vi "Shoot.vi"(1 "millisecond timer value":u32, 2 "Shoot":bool=TRUE) -> ()   [LabVIEW 2016]
uses:
  <vilib>/Rock Robotics/WPI/SafetyOutput/WPI_SafetyOutputConfigMenu.ctl
  Global 2.vi
  <vilib>/gmath/NI_Gmath.lvlib
panel:
  in  "Adjustment X":dbl[](array[numeric])=[-3400.0, -3100.0, -2750.0, -2430.0, -2080.0, -1710.0, -1330.0, -950.0, -580.0, -210.0, 0.0, 210.0, 580.0, 950.0, 1330.0, 1710.0, 2080.0, 2430.0, 2750.0, 3100.0, 3400.0]
  in  "Adjustment Y":dbl[](array[numeric])=[-1.0, -0.9, -0.8, -0.7, -0.6, -0.5, -0.4, -0.3, -0.2, -0.1, 0.0, 0.1, 0.2, 0.3, 0.4, 0.5, 0.6, 0.7, 0.8, 0.9, 1.0] format="%_6g"
  out "Waveform Chart":cluster{dbl}(graph)={2565.46875}
  out "Motor Effort":dbl=0.17108041660508766
  out "Adjustment":dbl=-0.27365642550017555
  out "RPM":dbl=2565.46875
  in  "kP":dbl=0.8 format="%#_13g"
  in  "kD":dbl=0.06 format="%#_13g"
  in  "Y":dbl[](array[numeric])=[0.0, 0.1, 0.2, 0.3, 0.4, 0.5, 0.6, 0.7, 0.8, 0.9, 1.0] format="%_6g"
  in  "X":dbl[](array[numeric])=[0.0, 210.0, 580.0, 950.0, 1330.0, 1710.0, 2080.0, 2430.0, 2750.0, 3100.0, 3400.0]
  in  "RPM Target BB":dbl=1500.0
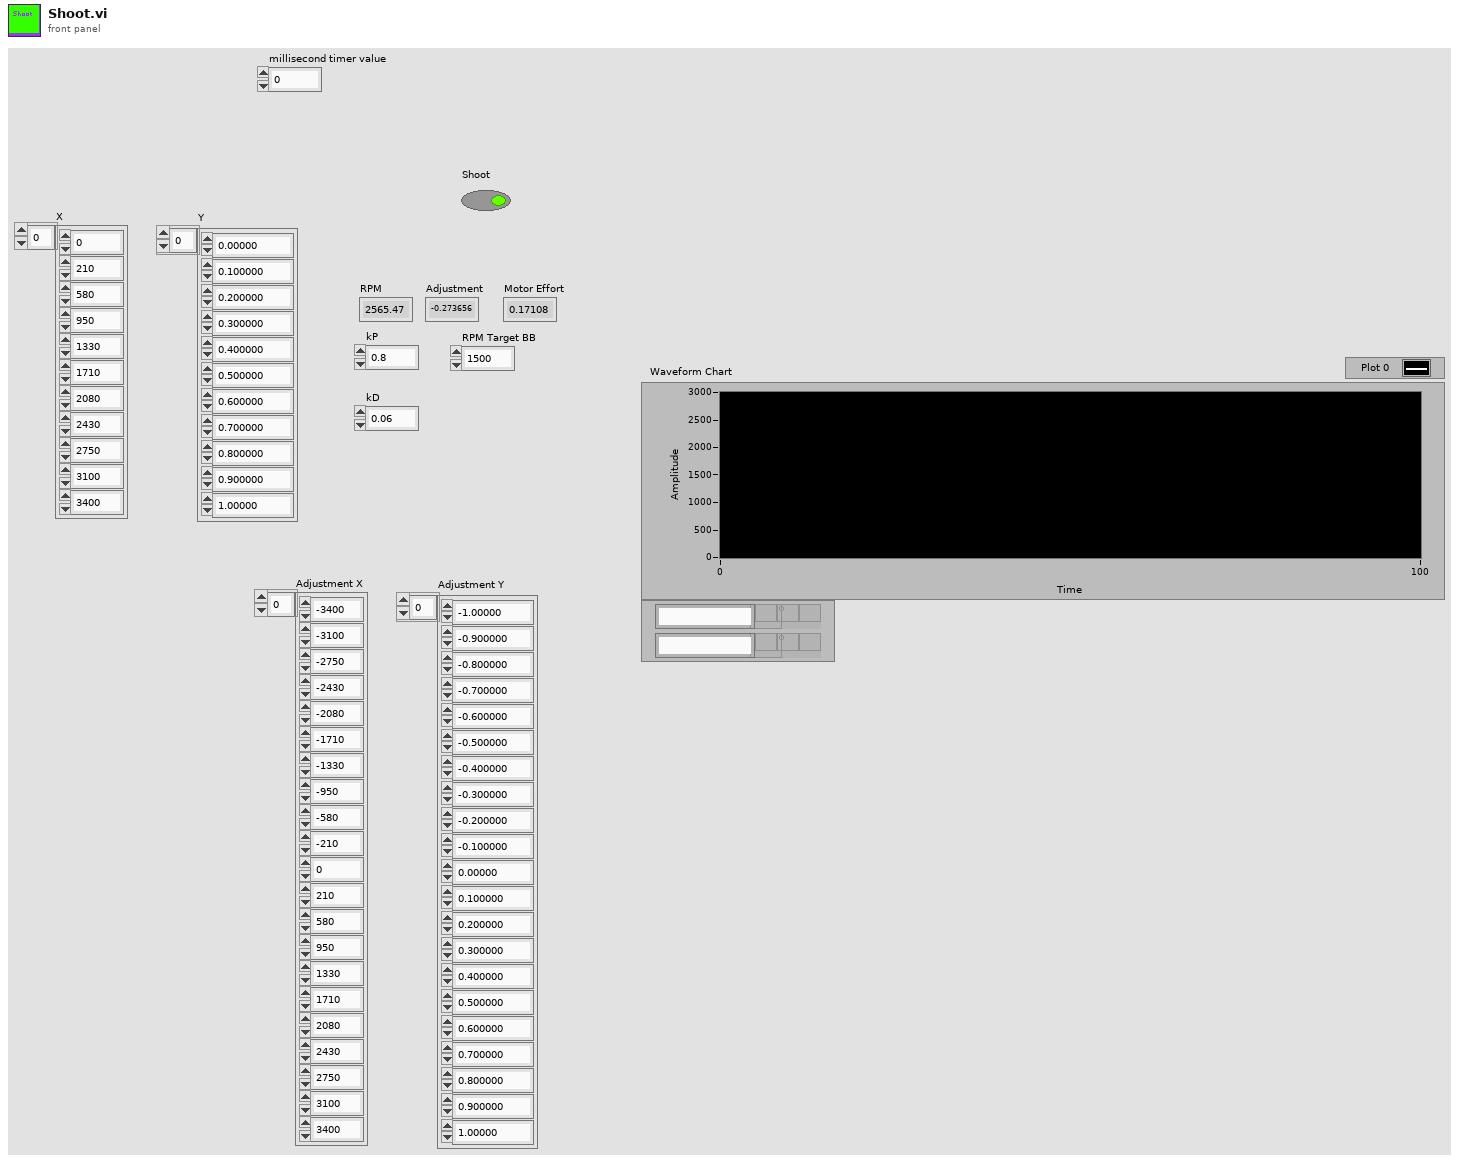
[diagram p1: front panel]
types:
  T1 = typedef "WPI_SafetyOutputConfigMenu.ctl" = enum16{"Enable", "Disable"}
  T2 = typedef "WPI_MotorControlDeviceRef.ctl" = cluster{"DeviceStatus":errorcluster, "Type":T3, "PWM":cluster{"PWM Channel":T4, "DeadBand":T5}, "CAN":cluster{"Device Number":u8, "SetOutput VI Ref":variant, "GetOutput VI Ref":variant, "Enable VI Ref":variant, "Disable VI Ref":variant, "Data":variant}, "Invert":bool}
  T3 = typedef "WPI_MotorControlType.ctl" = enum16{"PWM", "CAN"}
  T4 = typedef "FPGA_DIOPWMChannel.ctl" = enum8{"PWM 0", "PWM 1", "PWM 2", "PWM 3", "PWM 4", "PWM 5", "PWM 6", "PWM 7", "PWM 8", "PWM 9", "PWM MXP 0", "PWM MXP 1", "PWM MXP 2", "PWM MXP 3", "PWM MXP 4", "PWM MXP 5", "PWM MXP 6", "PWM MXP 7", "PWM MXP 8", "PWM MXP 9", "Invalid"}
  T5 = typedef "WPI_PWMDeadband.ctl" = cluster{"Name":string, "maxPositivePwm":i32, "minPositivePwm":i32, "centerPwm":i32, "maxNegativePwm":i32, "minNegativePwm":i32, "angularRange":u16}
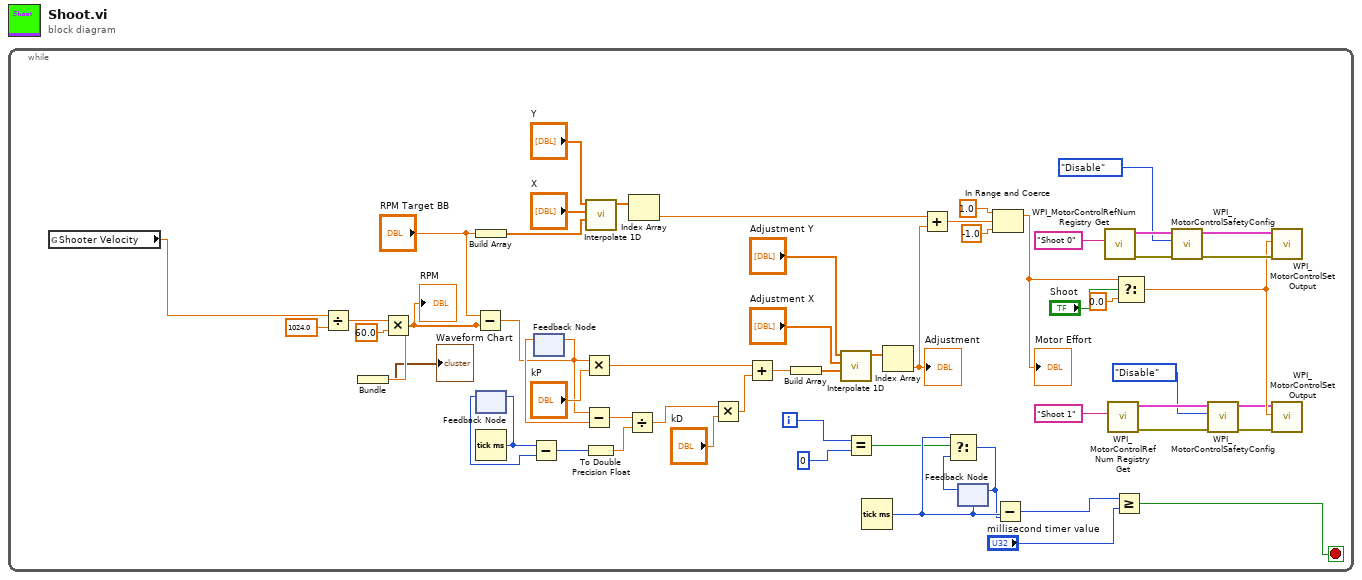
[diagram p0: block diagram]
diagram:
  n1 = while {
    i -> [w4]
    stop <- w1 stop-if-true
    n2 = global read "Global 2.vi" "Shooter Velocity"() -> (w21:dbl)
    n3 = Divide(x=w21, y=1024.0) -> (x/y=w56:dbl)
    n4 = Multiply(x=w56, y=60.0) -> (x*y=w27:dbl)
    "RPM" <- w27
    n5 = Bundle(w27) -> (→"Waveform Chart":cluster{dbl})  [unwired: 1 in]
    n6 = Subtract(x="RPM Target BB", y=w27) -> (x-y=w29:dbl)
    n7 = Build Array("RPM Target BB") -> (w54:dbl[])
    n8 = feedback #1() -> (w50:u32)  [unwired: 1 in]
    n9 = Tick Count (ms)() -> (millisecond timer value=w51:u32)
    n10 = feedback-in #1(w51) -> ()
    n11 = Subtract(x=w51, y=w50) -> (x-y=w48:u32)
    n12 = feedback #2() -> (w52:dbl)  [unwired: 1 in]
    n13 = feedback-in #2(w29) -> ()
    n14 = Multiply(x=w29, y="kP") -> (x*y=w42:dbl)
    n15 = Subtract(x=w29, y=w52) -> (x-y=w49:dbl)
    n16 = call <vilib>:"Interpolate 1D.vi"("xi"=w54, "X"="X", "Y"="Y") -> ("yi"=w53:dbl[])  [unwired: 6 in, 2 out]
    n17 = To Double Precision Float(number=w48) -> (double precision float=w47:dbl)
    n18 = Divide(x=w49, y=w47) -> (x/y=w46:dbl)
    n19 = Index Array(array=w53) -> (element=w40:dbl)  [unwired: 1 in]
    n20 = Multiply(x=w46, y="kD") -> (x*y=w41:dbl)
    n21 = Add(x=w42, y=w41) -> (x+y=w35:dbl)
    n22 = Build Array(w35) -> (w38:dbl[])
    n23 = call <vilib>:"Interpolate 1D.vi"("xi"=w38, "X"="Adjustment X", "Y"="Adjustment Y") -> ("yi"=w39:dbl[])  [unwired: 6 in, 2 out]
    n24 = Equal?(x=w4, y=0) -> (x = y?=w7:bool)
    n25 = Tick Count (ms)() -> (millisecond timer value=w9:u32)
    n26 = Index Array(array=w39) -> (element=w34:dbl)  [unwired: 1 in]
    "Adjustment" <- w34
    n27 = Add(x=w40, y=w34) -> (x+y=w33:dbl)
    n28 = feedback #3(w9) -> (w8:u32)
    n29 = Select(t=w9, s=w7, f=w8) -> (s? t:f=w5:u32)
    n30 = feedback-in #3(w5) -> ()
    n31 = In Range and Coerce(upper limit=1.0, x=w33, lower limit=-1.0 ("upper limit")) -> (coerced(x)=w30:dbl)  [unwired: 1 out]
    "Motor Effort" <- w30
    n32 = Subtract(x=w9, y=w5) -> (x-y=w3:u32)
    n33 = call <vilib>:"WPI_MotorControlRefNum Registry Get.vi"("refnum name"="Shoot 0") -> ("error out"=w10:errorcluster, "MotorControlDevRef"=w20:T2)  [unwired: 9 in]
    n34 = call <vilib>:"WPI_MotorControlRefNum Registry Get.vi"("refnum name"="Shoot 1") -> ("error out"=w15:errorcluster, "MotorControlDevRef"=w16:T2)  [unwired: 9 in]
    n35 = Greater Or Equal?(x=w3, y="millisecond timer value") -> (x >= y?=w1:bool)
    n36 = Select(t=w30, s="Shoot", f=0.0) -> (s? t:f=w14:dbl)
    n37 = call <vilib>:"WPI_MotorControlSafetyConfig.vi"("error in (no error)"=w10, "mode"=WPI_SafetyOutputConfigMenu."Disable", "MotorControlDevRef"=w20) -> ("error out"=w18:errorcluster, "MotorControlDevRef"=w19:T2)  [unwired: 7 in]
    n38 = call <vilib>:"WPI_MotorControlSafetyConfig.vi"("error in (no error)"=w15, "mode"=WPI_SafetyOutputConfigMenu."Disable", "MotorControlDevRef"=w16) -> ("error out"=w12:errorcluster, "MotorControlDevRef"=w13:T2)  [unwired: 7 in]
    n39 = call <vilib>:"WPI_MotorControlSetOutput.vi"("error in (no error)"=w18, "Output"=w14, "MotorControlDevRef"=w19) -> ()  [unwired: 6 in, 3 out]
    n40 = call <vilib>:"WPI_MotorControlSetOutput.vi"("error in (no error)"=w12, "Output"=w14, "MotorControlDevRef"=w13) -> ()  [unwired: 6 in, 3 out]
  }
